vi "Run Banana Configuration Tests.vi"() -> ()   [LabVIEW 2021]
uses:
  Bananas/Platano/Platano.lvclass
panel:
  out "error out":errorcluster
  out "Config Map":map{string, string}(c390)
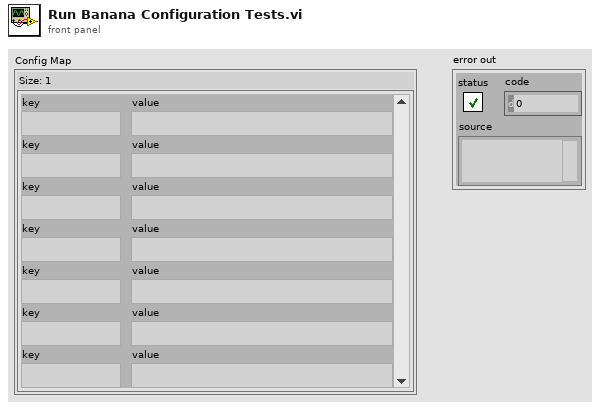
[diagram p1: front panel]
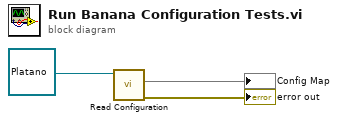
[diagram p0: block diagram]
diagram:
  n1 = call "Read Configuration.vi"("Platano in"=refnum<class "Platano.lvclass"> refnum ("Bananas.lvlib:Platano.lvclass")) -> ("error out"=→"error out":errorcluster, "Config Map"=→"Config Map":map{string, string})  [unwired: 8 in, 1 out]
